vi "pickVSSTeam.vi"(0 "Ally in":refnum<class "Ally.lvclass">, 1 "OldVSSTeam":refnum<class "Ally.lvclass">, 2 "RobotRef":refnum<class "Robot.lvclass">[](array[class]), 3 "error in (no error)":errorcluster, 4 "Game":refnum<class "Game.lvclass">) -> (7 "Ally out":refnum<class "Ally.lvclass">, 8 "RobotRef Out":refnum<class "Robot.lvclass">[](array[class]), 10 "error out":errorcluster)   [LabVIEW 2018, in "Ally.lvclass"]
uses:
  Ally.lvclass
  C:/Users/anton/Desktop/RoboIme/vsspssl/SSL_AI/Team_class/Team.lvclass
  Game_class/Game.lvclass
  Robot_class/Robot.lvclass
  Utilities_class/Utilities.lvclass
  Game_class/Game.lvclass/Game.ctl
  Team_class/Team.lvclass/Team.ctl
  Game_class/Read Parameters.lvclass.vi
  Team_class/Write RobotRef.vi
  Parameters_class/Parameters.lvclass
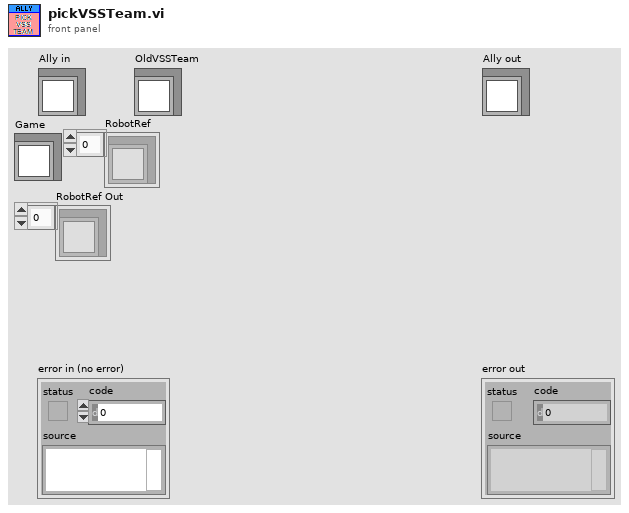
[diagram p1: front panel]
types:
  T1 = cluster{"Robots ids":cluster{"Goalie":enum16{"auto", "5", "4", "3", "2", "1", "0"}, "Attacker":enum16{"auto", "5", "4", "3", "2", "1", "0"}, "Defender":enum16{"auto", "5", "4", "3", "2", "1", "0"}}}
  T2 = cluster{"Goalie":enum16{"auto", "5", "4", "3", "2", "1", "0"}, "Attacker":enum16{"auto", "5", "4", "3", "2", "1", "0"}, "Defender":enum16{"auto", "5", "4", "3", "2", "1", "0"}}
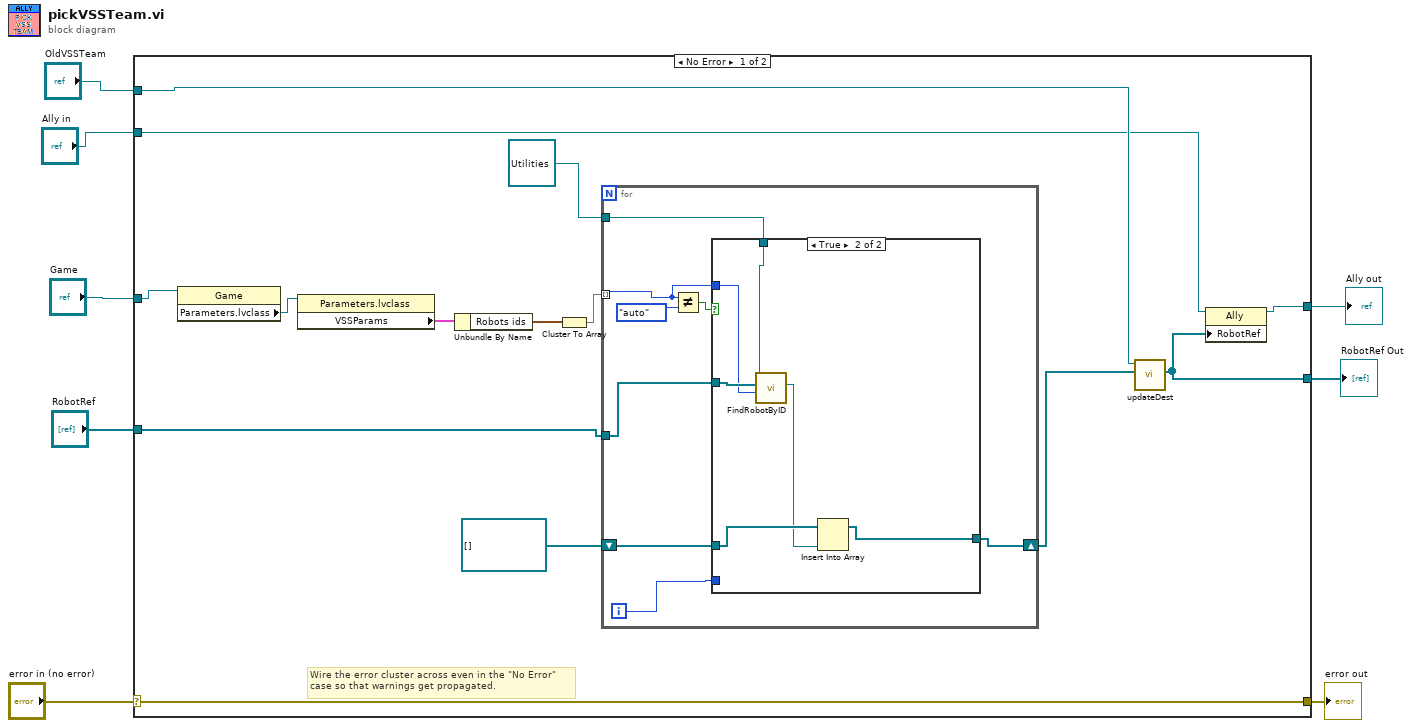
[diagram p0: block diagram]
diagram:
  n1 = case shown="No Error" "error in (no error)" {
    selector: "error in (no error)" -> [w22 w38]
    tunnel: [w22 w38] -> w7
    tunnel: "Game" -> [w21 _]
    tunnel: "OldVSSTeam" -> [w16 _]
    tunnel: "Ally in" -> [w15 _]
    tunnel: [w14 _] -> w3
    tunnel: [w13 _] -> w2
    tunnel: "RobotRef" -> [w12 _]
    frame No Error {
      # "Wire the error cluster across even in the \"No Error\"\ncase so that warnings get propagated."
      n2 = property class="Game"(reference=w21) -> ("Parameters.lvclass"=w20:refnum<class "Parameters.lvclass">)  [unwired: 1 in, 2 out]
      n3 = property class="Parameters.lvclass"(reference=w20) -> ("VSSParams"=w19:T1)  [unwired: 1 in, 2 out]
      n4 = Unbundle By Name(w19) -> ("Robots ids"=w17:T2)
      n5 = Cluster To Array(cluster=w17) -> (array=w18:enum16{"auto", "5", "4", "3", "2", "1", "0"}[])
      n6 = for {
        tunnel: w18 -> [w24] mode=indexing
        tunnel: w12 -> [w30]
        tunnel: refnum<class "Utilities.lvclass"> refnum ("Utilities in") -> [w29]
        shift-right: [w23] -> w9
        shift-left: refnum<class "Robot.lvclass">[] [] ("RobotRef") -> [w25]
        i -> [w26]
        n7 = Not Equal?(x=w24, y=enum16{"auto", "5", "4", "3", "2", "1", "0"}."auto") -> (x != y?=w27:bool)
        n8 = case shown="True" w27 {
          tunnel: w30 -> [_ w36]
          tunnel: w29 -> [_ w37]
          tunnel: [w31 w32] -> w23
          tunnel: w26 -> [_ _]
          tunnel: w25 -> [w31 w34]
          tunnel: w24 -> [_ w35]
          frame False {
          }
          frame True {
            n9 = call-dynamic "FindRobotByID.vi"("id"=w35, "RobotRef"=w36, "Utilities in"=w37) -> ("Robot"=w33:refnum<class "Robot.lvclass">)  [unwired: 5 in, 3 out]
            n10 = Insert Into Array(array=w34, new element=w33) -> (w32:refnum<class "Robot.lvclass">[])  [unwired: 1 in]
          }
        }
      }
      n11 = call "updateDest.vi"("NewAllyRobots"=w9, "LastAlly"=w16) -> ("NewAllyRobotsUpdated"=w13:refnum<class "Robot.lvclass">[])  [unwired: 7 in, 2 out]
      n12 = property class="Ally"(reference=w15, "RobotRef"=w13) -> (reference out=w14:refnum<class "Ally.lvclass">)  [unwired: 1 in, 1 out]
    }
    frame Error {
    }
  }
  "error out" <- w7
  "Ally out" <- w3
  "RobotRef Out" <- w2
